vi "Open Client Connection.vi"(8 "error in (no error)":errorcluster, 11 "RemoteControl.ZMQ in":refnum<class "RemoteControl.ZMQ.lvclass">) -> (0 "error out":errorcluster, 3 "RemoteControl.ZMQ out":refnum<class "RemoteControl.ZMQ.lvclass">)   [LabVIEW 2020, in "RemoteControl.ZMQ.lvclass"]
uses:
  RemoteControl.ZMQ.lvclass
  RemoteControl.ZMQ.lvclass/RemoteControl.ZMQ.ctl
  <vilib>/addons/zeromq/zmq_context.lvclass
  <vilib>/addons/zeromq/zmq_socket.lvclass
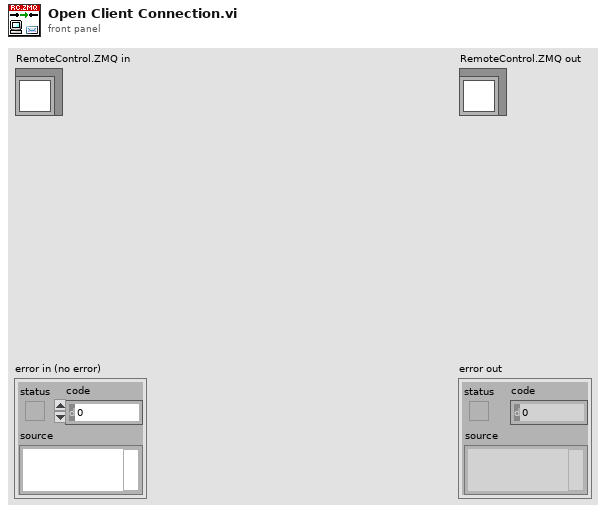
[diagram p1: front panel]
types:
  T1 = typedef "zeromq.lvlib/socket_type.ctl" = enum8{"ZMQ_PAIR", "ZMQ_PUB", "ZMQ_SUB", "ZMQ_REQ", "ZMQ_REP", "ZMQ_DEALER", "ZMQ_ROUTER", "ZMQ_PULL", "ZMQ_PUSH", "ZMQ_XPUB", "ZMQ_XSUB"}
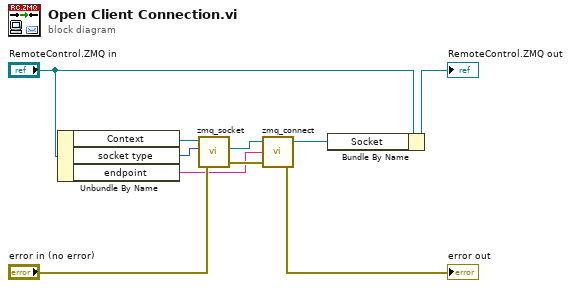
[diagram p0: block diagram]
diagram:
  n1 = Unbundle By Name("RemoteControl.ZMQ in") -> ("Context"=w8:refnum<class "zmq_context.lvclass">, "socket type"=w2:T1, "endpoint"=w1:string)
  n2 = call <vilib>:"zmq_socket.vi"("error in"="error in (no error)", "socket type"=w2, "context in"=w8) -> ("error out"=w4:errorcluster, "socket out"=w7:refnum<class "zmq_socket.lvclass">)  [unwired: 2 in, 1 out]
  n3 = call <vilib>:"zmq_connect.vi"("error in"=w4, "endpoint"=w1, "socket in"=w7) -> ("error out"=→"error out":errorcluster, "socket out"=w6:refnum<class "zmq_socket.lvclass">)  [unwired: 1 in]
  n4 = Bundle By Name(cluster="RemoteControl.ZMQ in", "Socket"=w6) -> (→"RemoteControl.ZMQ out":refnum<class "RemoteControl.ZMQ.lvclass">)
